vi "PFI-28000-System_Read Power Supply Voltage.vi"(0 "PFI-28000-System in":refnum<class "PFI-28000-System.lvclass">, 5 "Power Supply":T1, 11 "error in (no error)":errorcluster) -> (4 "PFI-28000-System out":refnum<class "PFI-28000-System.lvclass">, 6 "Voltage":dbl, 15 "error out":errorcluster)   [LabVIEW 2017, in "PFI-28000-System.lvclass"]
uses:
  PFI-28000-System.lvclass
  PFI-28000-System-Power Supply Select.ctl
  Utilities/PFI-28000-Utils.lvlib
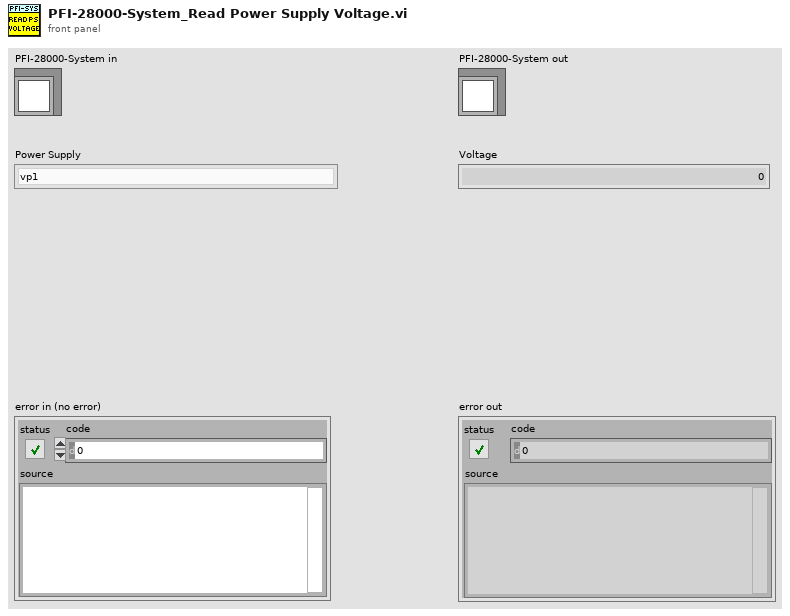
[diagram p1: front panel]
types:
  T1 = typedef "PFI-28000-System.lvclass/PFI-28000-System-Power Supply Select.ctl" = enum8{"vp1", "vp2", "vp3", "vp4", "vm1", "vm2", "vm3", "vm4", "+5vl", "viepe", "vfan"}
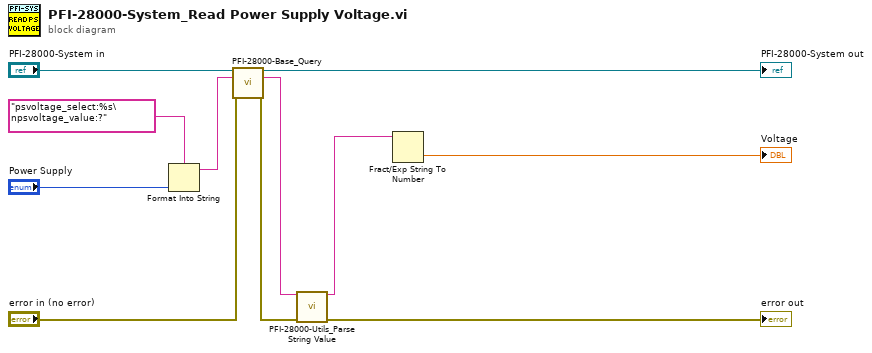
[diagram p0: block diagram]
diagram:
  n1 = Format Into String(format string="psvoltage_select:%s\npsvoltage_value:?" ("empty string"), "Power Supply") -> (resulting string=w8:string)  [unwired: 2 in, 1 out]
  n2 = call-dynamic "PFI-28000-Base_Query.vi"("PFI-28000-Base in"="PFI-28000-System in", "Command"=w8, "error in (no error)"="error in (no error)") -> ("PFI-28000-Base out"=→"PFI-28000-System out":refnum<class "PFI-28000-System.lvclass">, "Response"=w5:string, "error out"=w4:errorcluster)  [unwired: 9 in, 1 out]
  n3 = call "PFI-28000-Utils_Parse String Value.vi"("String"=w5, "error in (no error)"=w4) -> ("String Value"=w1:string, "error out"=→"error out":errorcluster)  [unwired: 11 in, 1 out]
  n4 = Fract/Exp String To Number(string=w1) -> (number=→"Voltage":dbl)  [unwired: 3 in, 1 out]
